vi "Split HDC Function Select.vi"(0 "IN 7:0":u8 format="%08b") -> (1 "OUT 1:0":fxp<+,2,2> format="%02b", 2 "OUT 7":bool, 3 "OUT 2":bool, 4 "OUT 3":bool, 5 "OUT 4":bool, 6 "OUT 5":bool)   [LabVIEW 2014]
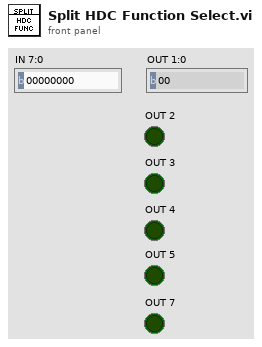
[diagram p1: front panel]
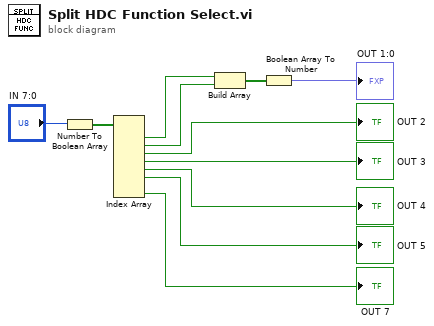
[diagram p0: block diagram]
diagram:
  n1 = Number To Boolean Array(number="IN 7:0") -> (Boolean array=w10:bool[])
  n2 = Index Array(array=w10) -> (element #1=w9:bool, element #2=w8:bool, element #3=→"OUT 2":bool, element #4=→"OUT 3":bool, element #5=→"OUT 4":bool, element #6=→"OUT 5":bool, element #8=→"OUT 7":bool)  [unwired: 8 in, 1 out]
  n3 = Build Array(w9, w8) -> (w7:bool[])
  n4 = Boolean Array To Number(Boolean array=w7) -> (number=→"OUT 1:0":fxp<+,2,2>)
